vi "Tension Solver.vi"(4 "QP?":bool=TRUE, 6 "P Gain":dbl[](array[numeric]), 7 "QP Stopping Criteria":T2={"function tolerance"=0.001, "parameter tolerance"=1e-05, "max iterations"=50, "max function calls"=50, "gradient tolerance"=1e-05, "max time (sec)"=0.01}, 9 "Reference X,Y":dbl[](array[numeric]), 10 "Measured Position":dbl[](array[numeric]), 11 "Motor Configuration":dbl[][](array[numeric])) -> (1 "Jacobian":T1, 2 "Reference Tension":dbl[](array[numeric]), 3 "QP Solved":bool=TRUE)   [LabVIEW 2021]
uses:
  <vilib>/gmath/NumericalOptimization/stopping criteria.ctl
  <vilib>/Analysis/Matrix/Datatypes/RealMatrix.ctl
  <vilib>/gmath/NI_Gmath.lvlib
  <vilib>/Analysis/Matrix/NI_Matrix.lvlib
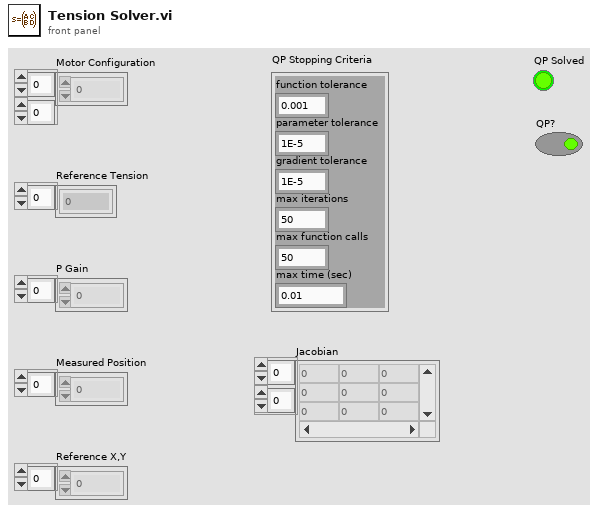
[diagram p1: front panel]
types:
  T1 = typedef "NI_Matrix.lvlib/RealMatrix.ctl" = dbl[][]
  T2 = typedef "NI_Gmath.lvlib/stopping criteria.ctl" = cluster{"function tolerance":dbl, "parameter tolerance":dbl, "max iterations":i32, "max function calls":i32, "gradient tolerance":dbl, "max time (sec)":dbl}
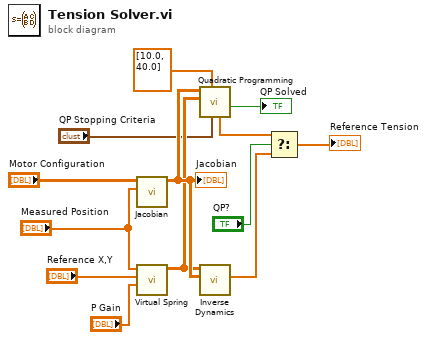
[diagram p0: block diagram]
diagram:
  n1 = call "Jacobian.vi"("EE Position"="Measured Position", "Motor Configuration"="Motor Configuration") -> ("Jacobian"=w12:T1)  [unwired: 9 in]
  "Jacobian" <- w12
  n2 = call "Virtual Spring.vi"("P Gain"="P Gain", "Reference Position"="Reference X,Y", "Actual Position"="Measured Position") -> ("Desired Force Matrix"=w2:T1)  [unwired: 8 in]
  n3 = call "Quadratic Programming.vi"("stopping Criteria"="QP Stopping Criteria", "UB"=dbl[] [10.0, 40.0] ("LB"), "Desired Force Matrix"=w2, "Jacobian"=w12) -> ("Boolean"=→"QP Solved":bool, "minimum"=w4:dbl[])  [unwired: 4 in, 2 out]
  n4 = call "Inverse Dynamics.vi"("Jacobian Matrix"=w12, "F desired Matrix"=w2) -> ("Reference Tension"=w3:dbl[])  [unwired: 9 in]
  n5 = Select(t=w4, s="QP?", f=w3) -> (s? t:f=→"Reference Tension":dbl[])
